vi "Mode (Read).vi"(6 "ISOBUS address":T3=-1 caption="ISOBUS address (-1)", 8 "error in":errorcluster, 11 "Mercury Reference In":T4) -> (0 "error out":errorcluster, 2 "Mode":T1="NORM" caption="User Mode", 3 "Mercury Reference Out":T4, 4 "Valid?":T2)   [LabVIEW 2013, in "Mercury iXX.lvlib" / "System.lvlib"]
doc: "Returns the current user mode according to the instrument."
uses:
  <instrlib>/Mercury iXX/Public/Libraries/System.lvlib
  <instrlib>/Mercury iXX/Public/Controls/Mercury Reference.ctl
  <instrlib>/Mercury iXX/Public/Controls/Comms Transport Layer.ctl
  <instrlib>/Mercury iXX/Private/Controls/Query Dynamic Reference.ctl
  <instrlib>/Mercury iXX/Public/Controls/ISOBus Address.ctl
  <instrlib>/Mercury iXX/Public/Controls/Is Valid LED.ctl
  <instrlib>/Mercury iXX/Public/Libraries/System/Controls/User Mode.ctl
  <instrlib>/Mercury iXX/Private/Controls/Command Verbs.ctl
  <instrlib>/Mercury iXX/Mercury iXX.lvlib
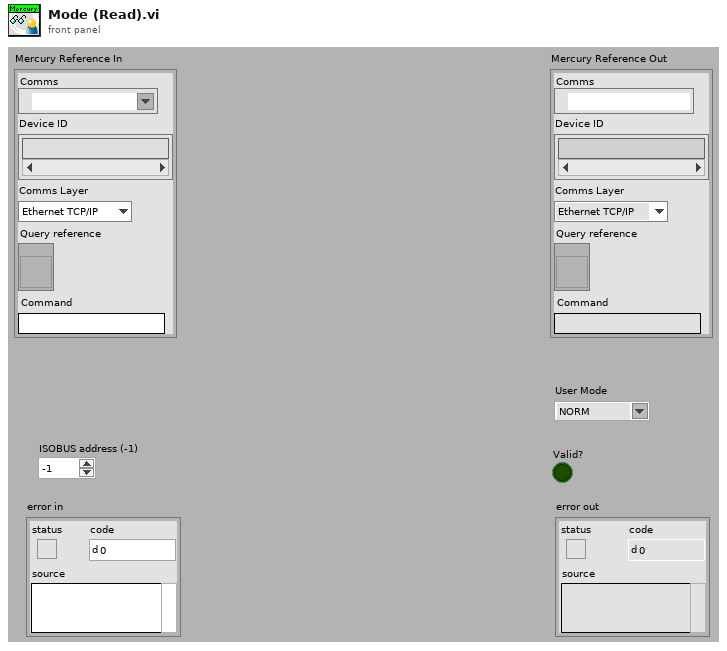
[diagram p1: front panel]
types:
  T1 = typedef "Mercury iXX.lvlib/System.lvlib/User Mode.ctl" = string
  T2 = typedef "Mercury iXX.lvlib/Is Valid LED.ctl" = bool
  T3 = typedef "Mercury iXX.lvlib/ISOBus Address.ctl" = i32
  T4 = typedef "Mercury iXX.lvlib/Mercury Reference.ctl" = cluster{"Comms":refnum<visa-resource-name>, "Device ID":string[], "Comms Layer":T5, "Command":string, "Query reference":T6}
  T5 = typedef "Mercury iXX.lvlib/Comms Transport Layer.ctl" = enum16{"Ethernet TCP/IP", "USB", "ISOBus - RS-232", "GPIB"}
  T6 = typedef "Mercury iXX.lvlib/Query Dynamic Reference.ctl" = refnum<vi>
  T7 = typedef "Mercury iXX.lvlib/Command Verbs.ctl" = string
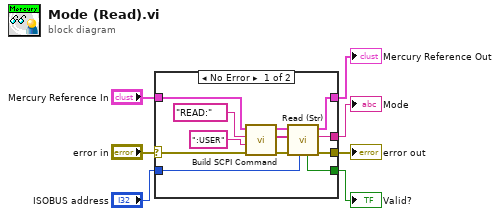
[diagram p0: block diagram]
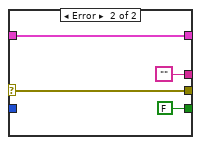
[diagram p2: hidden frame]
diagram:
  n1 = case shown="No Error" "error in" {
    selector: "error in" -> [w11 w22]
    tunnel: "Mercury Reference In" -> [w13 w23]
    tunnel: [w19 w23] -> w6
    tunnel: [w18 w22] -> w5
    tunnel: "ISOBUS address" -> [w17 _]
    tunnel: [w15 ""] -> w1
    tunnel: [w16 FALSE ("Valid?")] -> w2
    frame No Error {
      n2 = call <instrlib>:"Build SCPI Command.vi"("error in"=w11, "Noun(s)"=":USER" ("Command"), "Verb"=T7 "READ:", "Mercury Reference In"=w13) -> ("error out"=w10:errorcluster, "SCPI Message(s)"=w9:string[], "Mercury Reference Out"=w12:T4)  [unwired: 5 out]
      n3 = call <instrlib>:"Read (Str).vi"("ISOBUS address"=w17, "error in"=w10, "SCPI Message(s)"=w9, "Mercury Reference In"=w12) -> ("error out"=w18:errorcluster, "Response"=w15:string, "Mercury Reference Out"=w19:T4, "Valid?"=w16:T2)  [unwired: 4 out]
    }
    frame Error {
    }
  }
  "Mercury Reference Out" <- w6
  "error out" <- w5
  "Valid?" <- w2
  "Mode" <- w1
